vi "BRig_dataExp_CueSwitch_PreR.vi"() -> (2 "output_CueSwitch_PreR":i32)   [LabVIEW 2014]
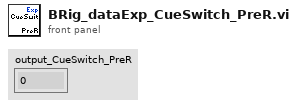
[diagram p1: front panel]
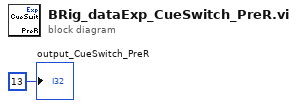
[diagram p0: block diagram]
diagram:
  "output_CueSwitch_PreR" <- 13 ("output_iBlock")
